vi "Example-ITC.vi"() -> ()   [LabVIEW 2013, in "Mercury iXX.lvlib"]
uses:
  <instrlib>/Mercury iXX/Mercury iXX.lvlib
  <instrlib>/Mercury iXX/Public/Controls/Unit String.ctl
  <instrlib>/Mercury iXX/Public/Libraries/Temperature/Controls/Temperature Device (Read).ctl
  <instrlib>/Mercury iXX/Public/Controls/Manufacturing Data.ctl
  <instrlib>/Mercury iXX/Public/Libraries/Temperature/Controls/Temperature Sensor Type.ctl
  <instrlib>/Mercury iXX/Public/Libraries/Temperature/Controls/Excitation Cluster.ctl
  <instrlib>/Mercury iXX/Public/Libraries/Temperature/Controls/Excitation Type.ctl
  <instrlib>/Mercury iXX/Public/Libraries/Temperature/Controls/Calibration Cluster.ctl
  <instrlib>/Mercury iXX/Public/Libraries/Temperature/Controls/Calibration Interpolation.ctl
  <instrlib>/Mercury iXX/Public/Libraries/Temperature/Controls/Loop Cluster.ctl
  <instrlib>/Mercury iXX/Public/Libraries/Temperature/Controls/Temperature Signals Cluster.ctl
  <instrlib>/Mercury iXX/Public/Libraries/Heater/Controls/Heater Device (Read).ctl
  <instrlib>/Mercury iXX/Public/Libraries/Heater/Controls/Heater Signals Cluster.ctl
  <instrlib>/Mercury iXX/Public/Libraries/Auxiliary/Controls/AUX Device (Read).ctl
  <instrlib>/Mercury iXX/Public/Libraries/Auxiliary/Controls/AUX Signals (Read).ctl
  <instrlib>/Mercury iXX/Public/Libraries/Pressure/Controls/Pressure Device (Read).ctl
  <instrlib>/Mercury iXX/Public/Libraries/Pressure/Controls/Pressure Sensor Type.ctl
  <instrlib>/Mercury iXX/Public/Libraries/Pressure/Controls/Calibration Cluster.ctl
  <instrlib>/Mercury iXX/Public/Libraries/Pressure/Controls/Calibration Interpolation.ctl
  <instrlib>/Mercury iXX/Public/Libraries/Pressure/Controls/Loop Cluster.ctl
  <instrlib>/Mercury iXX/Public/Libraries/Pressure/Controls/Pressure Signals Cluster.ctl
  <instrlib>/Mercury iXX/Public/Libraries/Flow/Controls/Flow Device (Read).ctl
  <instrlib>/Mercury iXX/Public/Libraries/Flow/Controls/Flow Signals Cluster.ctl
  <instrlib>/Mercury iXX/Public/Controls/Comms Transport Layer.ctl
  <instrlib>/Mercury iXX/Public/Controls/ISOBus Address.ctl
  <instrlib>/Mercury iXX/Public/Libraries/System/Open/Open System.vi
  <instrlib>/Mercury iXX/Public/Libraries/System/Read/Catalogue (Read).vi
  <instrlib>/Mercury iXX/Public/Libraries/System/Read/Display Automatic Dimming (Read).vi
  <instrlib>/Mercury iXX/Public/Libraries/System/Read/Display Automatic Dimming Time (Read).vi
  <instrlib>/Mercury iXX/Public/Libraries/System/Read/Display Brightness (Read).vi
  <instrlib>/Mercury iXX/Public/Libraries/System/Read/Date (Read).vi
  <instrlib>/Mercury iXX/Public/Libraries/System/Read/Time (Read).vi
  <instrlib>/Mercury iXX/Public/Libraries/System/Read/DateTime (Read).vi
  <instrlib>/Mercury iXX/Public/Libraries/System/Read/HVer (Read).vi
  <instrlib>/Mercury iXX/Public/Libraries/System/Read/FVer (Read).vi
  <instrlib>/Mercury iXX/Public/Libraries/System/Read/Serial Number (Read).vi
  <instrlib>/Mercury iXX/Public/Libraries/System/Read/Flash Space (Read).vi
  <instrlib>/Mercury iXX/Public/Libraries/System/Read/Mode (Read).vi
  <instrlib>/Mercury iXX/Public/Libraries/Auxiliary/Open/Open Auxiliary Device.vi
  <instrlib>/Mercury iXX/Public/Libraries/Auxiliary/Configuration/Read/Aux Device (Read).vi
  <instrlib>/Mercury iXX/Public/Libraries/Auxiliary/Configuration/Read/Serial Number (Read).vi
  <instrlib>/Mercury iXX/Public/Libraries/Auxiliary/Configuration/Read/Minimum Gas Flow (Read).vi
  <instrlib>/Mercury iXX/Public/Libraries/Auxiliary/Configuration/Read/Gas Flow Scaling (Read).vi
  <instrlib>/Mercury iXX/Public/Libraries/Auxiliary/Configuration/Read/Temperature Error Sensitivity (Read).vi
  <instrlib>/Mercury iXX/Public/Libraries/Auxiliary/Configuration/Read/Temperature Error Voltage Sensitivity (Read).vi
  <instrlib>/Mercury iXX/Public/Libraries/Auxiliary/Configuration/Read/Valve Gearing (Read).vi
  <instrlib>/Mercury iXX/Public/Libraries/Auxiliary/Configuration/Read/Stepper Speed (Read).vi
  <instrlib>/Mercury iXX/Public/Libraries/Auxiliary/Signals/Read/Position (Read).vi
  <instrlib>/Mercury iXX/Public/Libraries/Auxiliary/Signals/Read/Percent Open (Read).vi
  <instrlib>/Mercury iXX/Public/Libraries/Pressure/Open/Open Pressure Device.vi
  <instrlib>/Mercury iXX/Public/Libraries/Pressure/Configuration/Read/Pressure Device (Read).vi
  <instrlib>/Mercury iXX/Public/Libraries/Pressure/Configuration/Read/Nickname (Read).vi
  <instrlib>/Mercury iXX/Public/Libraries/Pressure/Signals/Read/Current (Read).vi
  <instrlib>/Mercury iXX/Public/Libraries/Pressure/Signals/Read/Voltage (Read).vi
  <instrlib>/Mercury iXX/Public/Libraries/Heater/Open/Open Heater Device.vi
  <instrlib>/Mercury iXX/Public/Libraries/Heater/Configuration/Read/Heater Device (Read).vi
  <instrlib>/Mercury iXX/Public/Libraries/Heater/Configuration/Read/Nickname (Read).vi
  <instrlib>/Mercury iXX/Public/Libraries/Heater/Configuration/Read/Serial Number (Read).vi
  <instrlib>/Mercury iXX/Public/Libraries/Heater/Configuration/Read/Voltage Limit (Read).vi
  <instrlib>/Mercury iXX/Public/Libraries/Heater/Configuration/Read/Nominal Resistance (Read).vi
  <instrlib>/Mercury iXX/Public/Libraries/Heater/Configuration/Read/Maximum Power (Read).vi
  <instrlib>/Mercury iXX/Public/Libraries/Heater/Signals/Read/Voltage (Read).vi
  <instrlib>/Mercury iXX/Public/Libraries/Heater/Signals/Read/Power (Read).vi
  <instrlib>/Mercury iXX/Public/Libraries/Heater/Signals/Read/Current (Read).vi
  <instrlib>/Mercury iXX/Public/Libraries/Temperature/Open/Open Temperature Device.vi
  <instrlib>/Mercury iXX/Public/Libraries/Temperature/Configuration/Read/Serial Number (Read).vi
  <instrlib>/Mercury iXX/Public/Libraries/Temperature/Configuration/Read/Nickname (Read).vi
  <instrlib>/Mercury iXX/Public/Libraries/Temperature/Configuration/Read/Excitation Magnitude (Read).vi
  <instrlib>/Mercury iXX/Public/Libraries/Temperature/Configuration/Read/Temperature Sensor (Read).vi
  <instrlib>/Mercury iXX/Public/Libraries/Temperature/Configuration/Read/Excitation Type (Read).vi
  <instrlib>/Mercury iXX/Public/Libraries/Temperature/Configuration/Read/Calibration Hot Limit (Read).vi
  <instrlib>/Mercury iXX/Public/Libraries/Temperature/Configuration/Read/Calibration Cold Limit (Read).vi
  <instrlib>/Mercury iXX/Public/Libraries/Temperature/Signals/Read/Temperature (Read).vi
  <instrlib>/Mercury iXX/Public/Libraries/Temperature/Configuration/Read/Temperature Device (Read).vi
  <instrlib>/Mercury iXX/Public/Libraries/Control Loop/Configuration/Read/Control Loop (Read).vi
  <instrlib>/Mercury iXX/Public/Libraries/System/Set/DateTime (Set).vi
  <instrlib>/Mercury iXX/Public/Libraries/Pressure.lvlib
  <instrlib>/Mercury iXX/Public/Libraries/System.lvlib
  <instrlib>/Mercury iXX/Public/Libraries/Auxiliary.lvlib
  <instrlib>/Mercury iXX/Public/Libraries/Control Loop.lvlib
  <instrlib>/Mercury iXX/Public/Libraries/Heater.lvlib
  <instrlib>/Mercury iXX/Public/Libraries/Temperature.lvlib
  <instrlib>/Mercury iXX/Public/Libraries/Flow/Open/Open Flow Device.vi
  <instrlib>/Mercury iXX/Public/Libraries/Flow.lvlib
  <instrlib>/Mercury iXX/Public/Libraries/Flow/Configuration/Read/Flow Device (Read).vi
  <instrlib>/Mercury iXX/Public/Libraries/Flow/Configuration/Read/Maximum Power (Read).vi
  <instrlib>/Mercury iXX/Public/Libraries/Flow/Configuration/Read/Fastcool Mode (Read).vi
  <instrlib>/Mercury iXX/Public/Libraries/Flow/Signals/Read/Voltage (Read).vi
  <instrlib>/Mercury iXX/Public/Libraries/Flow/Signals/Read/Current (Read).vi
panel:
  in  "Mercury Functions":T1(tab)
  out "time stamp":timestamp=timestamp(3542718986 s since 1904-01-01)
  out "Free Space":i32=166152 caption="Free Space (KB)"
  out "Set Date Response":string="VALID"
  out "String":string="NORM" caption="User Mode"
  out "Date":string="2016:04:05"
  out "Time":string="11:36:26"
  out "Hardware Version":string="65"
  out "Firmware Version":string="2.2.6.20"
  out "Serial Number":string="153350063"
  out "Devices":string[](array[string])=["DB3.L1:LVL", "GRPX:PSU", "GRPY:PSU", "GRPZ:PSU", "MB1.T1:TEMP", "PSU.M1:PSU", "PSU.M2:PSU", "PSU.M3:PSU"]
  out "S/W Version(s)":string[](array[string])=["2.2.6.20\n"]
  out "Serial Number(s)":string[](array[string])=["153350063"]
  out "# of Instruments":i32=1
  out "Automatic Dimming":string="OFF"
  out "Dimming Time":string="5"
  out "Display Brightness":string="100"
  in  "ITC IP Address":string="130.49.180.102"
  out "Excitation Magnitude":dbl
  out "Sensor Type":string="DUM"
  out "Excitation Type":string="UNIP"
  out "Hot Limit":dbl=1000.0
  out "H Unit":T2="K"
  out "Cold Limit":dbl=1000.0
  out "C Unit":T2="K"
  out "Unit":T2
  out "Voltage":dbl
  out "V Unit":T2="A"
  out "Temperature":dbl
  out "T Unit":T2="K"
  out "Temperature Device Settings":T3={"Manufacturing"={"Hardware Version"="65", "Firmware Version"="2.2", "Serial Number"="153350063"}, "Temperature Sensor Type"="DUM", "Excitation"={"Excitation Type"="UNIP", "Magnitude"="0"}, "Calibration"={"Filename"="None", "Interpolation"="LIN", "Scaling Factor"="1", "Offset Factor"="0", "Hot Limit"="1000.00K", "Cold Limit"="1000.00K", "Last Calibration"="", "Reference"="Internal"}, "Control Loop"={"Heater"="", "Auxiliary"="", "Heater Auto"="", "Percentage Heat"="", "Temperature Set Point"="", "PID Auto (from file)"="", "P Value"="", "I Value"="", "D Value"="", "Auto PID Table Filename"="", "Flow Auto"="", "Target Heater Table"="", "Sweep mode"="", "Sweep Table Filename"="", "Percentage Flow"=""}, "Temperature Signals"={"Voltage"="0.0000V", "Current"="0.0000A", "Power"="N/A", "Resistance"="", "Temperature"="0.0000K", "Sensitivity"="", "Reference"=""}, "Nickname"="MB1.T1", "Status"="0"}
  out "Temp S/N":string="153350063"
  out "T Nickname":string="MB1.T1"
  out "T Loop Details":T10
  out "Heater Device Settings":T12={"Manufacturing"={"Hardware Version"="", "Firmware Version"="", "Serial Number"=""}, "Nickname"="", "Voltage Limit"="", "Nominal Resistance"="", "Maximum Power"="", "Heater Signals"={"Voltage"="", "Current"="", "Power"=""}, "Status"="DEV"}
  out "Htr C Unit":T2
  out "Htr P Unit":T2
  out "Htr V Unit":T2
  out "Htr Current":dbl
  out "Htr Power":dbl
  out "Htr Voltage":dbl
  out "Power Unit":T2
  out "Volt Unit":T2
  out "Res Unit":T2
  out "Maximum Power":dbl
  out "Htr Resistance":dbl
  out "Htr Voltage Limit":dbl
  out "Htr S/N":string="STAT:DEV:MB0.H1:N/A"
  out "Htr Nickname":string="STAT:DEV:MB0.H1:N/A"
  out "Auxiliary Device Details":T14 {"Signals"."% Open" min=0.0 max=100.0 step=0.1 format="%.4f"; "Signals"."Position" max=20.0 step=1.0 format="%.4f"; "Speed" max=7 step=1; "Gear" max=7 step=1; "Temp V Err" min=0.0 max=20.0 step=0.1; "Temp Err" min=0.0 max=20.0 step=0.1; "Scaling Factor" min=0.0 max=99.0 step=0.1; "Min Flow" min=0.0 max=20.0 step=0.1}
  out "Aux S/N":string
  out "Min Flow":dbl=-inf caption="Minimum Gas Flow" format="%#.1f"
  out "Scaling Factor":dbl=-inf caption="Gas Flow Scaling Factor" format="%#.1f"
  out "Temp Err":dbl=-inf caption="Temperature Error Sensitivity" format="%#.1f"
  out "Temp V Err":dbl=-inf caption="Temperature Voltage Error Sensitivity" format="%#.1f"
  out "Gear":u32 caption="Valve Gearing"
  out "Speed":u32 caption="Stepper Speed"
  out "Unit 2":T2="ERR"
  out "Unit 3":T2="ERR"
  out "Unit 4":T2="ERR"
  out "Unit 5":T2="ERR"
  out "Unit 6":T2="ERR"
  out "Unit 7":T2="ERR"
  out "Position":u32
  out "% Open":dbl=-inf caption="Percentage Open (%)"
  out "Unit":T2="ERR"
  out "Unit":T2="ERR"
  out "Pressure Device":T16={"Manufacturing"={"Hardware Version"="", "Firmware Version"="", "Serial Number"=""}, "Temperature Sensor Type"="", "Calibration"={"Filename"="", "Interpolation"="", "Scaling Factor"="", "Offset Factor"="", "High Limit"="", "Low Limit"="", "Last Calibration"=""}, "Control Loop"={"Heater"="", "Auxiliary"="", "Heater Auto"="", "Percentage Heat"="", "Pressure Set Point"="", "PID Auto (from file)"="", "P Value"="", "I Value"="", "D Value"="", "Auto PID Table Filename"="", "Flow Auto"="", "Target Heater Table"="", "Sweep mode"="", "Sweep Table Filename"="", "Percentage Flow"=""}, "Pressure Signals"={"Voltage"="", "Current"="", "Power"="", "Pressure"=""}, "Nickname"="", "Status"="DEV"}
  out "Nickname":string="STAT:DEV:DB6.P1:N/A"
  out "Current":dbl
  out "Voltage":dbl
  out "Flow Device":T22
  out "Maximum Power 2":dbl
  out "Fastcool Mode":string
  out "Current 2":dbl
  out "Voltage 2":dbl
  # "ITC"
  # "101, 102, 67"
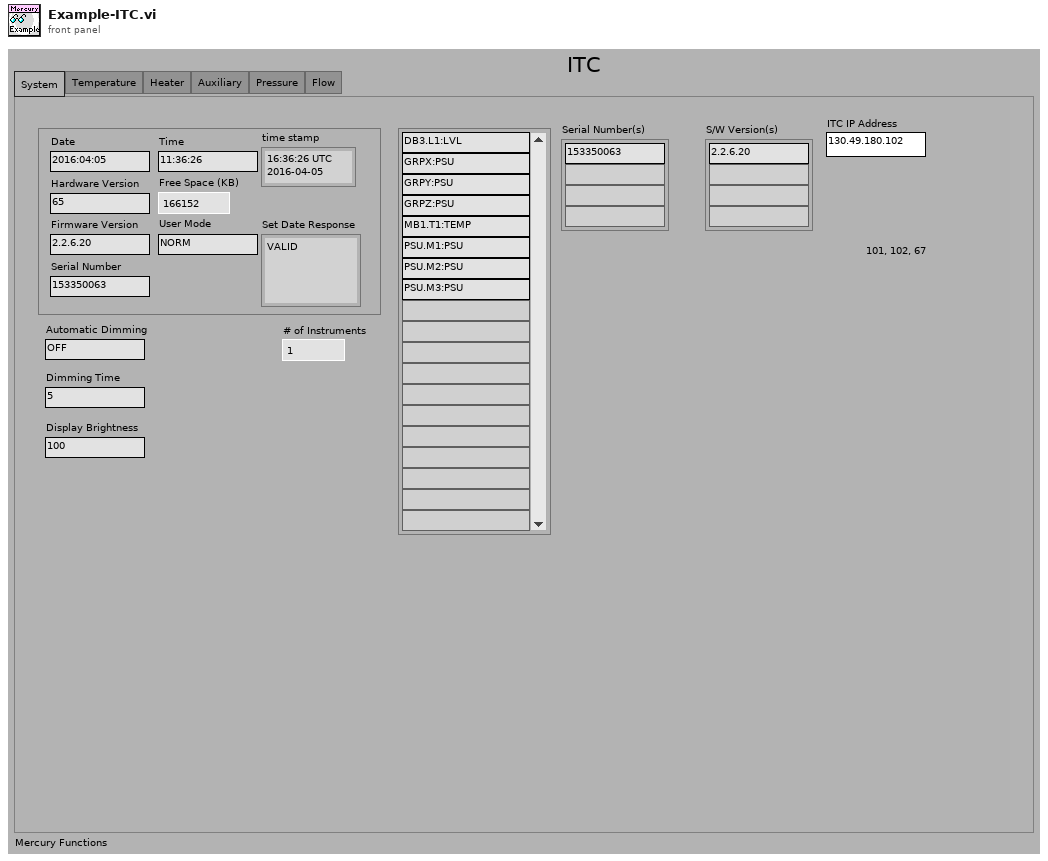
[diagram p1: front panel]
types:
  T1 = enum32{"System", "Temperature", "Heater", "Auxiliary", "Pressure", "Flow"}
  T2 = typedef "Mercury iXX.lvlib/Unit String.ctl" = string
  T3 = typedef "Mercury iXX.lvlib/Temperature.lvlib/Temperature Device (Read).ctl" = cluster{"Manufacturing":T4, "Temperature Sensor Type":T5, "Excitation":T6, "Calibration":T8, "Control Loop":T10, "Temperature Signals":T11, "Nickname":string, "Status":string}
  T4 = typedef "Mercury iXX.lvlib/Manufacturing Data.ctl" = cluster{"Hardware Version":string, "Firmware Version":string, "Serial Number":string}
  T5 = typedef "Mercury iXX.lvlib/Temperature.lvlib/Temperature Sensor Type.ctl" = string
  T6 = typedef "Mercury iXX.lvlib/Temperature.lvlib/Excitation Cluster.ctl" = cluster{"Excitation Type":T7, "Magnitude":string}
  T7 = typedef "Mercury iXX.lvlib/Temperature.lvlib/Excitation Type.ctl" = string
  T8 = typedef "Mercury iXX.lvlib/Temperature.lvlib/Calibration Cluster.ctl" = cluster{"Filename":string, "Interpolation":T9, "Scaling Factor":string, "Offset Factor":string, "Hot Limit":string, "Cold Limit":string, "Last Calibration":string, "Reference":string}
  T9 = typedef "Mercury iXX.lvlib/Temperature.lvlib/Calibration Interpolation.ctl" = string
  T10 = typedef "Mercury iXX.lvlib/Temperature.lvlib/Loop Cluster.ctl" = cluster{"Heater":string, "Auxiliary":string, "Heater Auto":string, "Percentage Heat":string, "Temperature Set Point":string, "PID Auto (from file)":string, "P Value":string, "I Value":string, "D Value":string, "Auto PID Table Filename":string, "Flow Auto":string, "Target Heater Table":string, "Sweep mode":string, "Sweep Table Filename":string, "Percentage Flow":string}
  T11 = typedef "Mercury iXX.lvlib/Temperature.lvlib/Temperature Signals Cluster.ctl" = cluster{"Voltage":string, "Current":string, "Power":string, "Resistance":string, "Temperature":string, "Sensitivity":string, "Reference":string}
  T12 = typedef "Mercury iXX.lvlib/Heater.lvlib/Heater Device (Read).ctl" = cluster{"Manufacturing":T4, "Nickname":string, "Voltage Limit":string, "Nominal Resistance":string, "Maximum Power":string, "Heater Signals":T13, "Status":string}
  T13 = typedef "Mercury iXX.lvlib/Heater.lvlib/Heater Signals Cluster.ctl" = cluster{"Voltage":string, "Current":string, "Power":string}
  T14 = typedef "Mercury iXX.lvlib/Auxiliary.lvlib/AUX Device (Read).ctl" = cluster{"Manufacturing":T4, "Min Flow":dbl, "Scaling Factor":dbl, "Temp Err":dbl, "Temp V Err":dbl, "Gear":u32, "Speed":u32, "Signals":T15, "Nickname":string, "Status":string}
  T15 = typedef "Mercury iXX.lvlib/Auxiliary.lvlib/AUX Signals (Read).ctl" = cluster{"Position":dbl, "% Open":dbl, "I0":string, "I1":string, "I2":string, "I3":string, "O0":string, "O1":string, "O2":string, "O3":string}
  T16 = typedef "Mercury iXX.lvlib/Pressure.lvlib/Pressure Device (Read).ctl" = cluster{"Manufacturing":T4, "Temperature Sensor Type":T17, "Calibration":T18, "Control Loop":T20, "Pressure Signals":T21, "Nickname":string, "Status":string}
  T17 = typedef "Mercury iXX.lvlib/Pressure.lvlib/Pressure Sensor Type.ctl" = string
  T18 = typedef "Mercury iXX.lvlib/Pressure.lvlib/Calibration Cluster.ctl" = cluster{"Filename":string, "Interpolation":T19, "Scaling Factor":string, "Offset Factor":string, "High Limit":string, "Low Limit":string, "Last Calibration":string}
  T19 = typedef "Mercury iXX.lvlib/Pressure.lvlib/Calibration Interpolation.ctl" = string
  T20 = typedef "Mercury iXX.lvlib/Pressure.lvlib/Loop Cluster.ctl" = cluster{"Heater":string, "Auxiliary":string, "Heater Auto":string, "Percentage Heat":string, "Pressure Set Point":string, "PID Auto (from file)":string, "P Value":string, "I Value":string, "D Value":string, "Auto PID Table Filename":string, "Flow Auto":string, "Target Heater Table":string, "Sweep mode":string, "Sweep Table Filename":string, "Percentage Flow":string}
  T21 = typedef "Mercury iXX.lvlib/Pressure.lvlib/Pressure Signals Cluster.ctl" = cluster{"Voltage":string, "Current":string, "Power":string, "Pressure":string}
  T22 = typedef "Mercury iXX.lvlib/Flow.lvlib/Flow Device (Read).ctl" = cluster{"Manufacturing":T4, "Nickname":string, "Voltage Limit":string, "Nominal Resistance":string, "Maximum Power":string, "Flow Signals":T23, "Status":string, "Fastcool Mode":string}
  T23 = typedef "Mercury iXX.lvlib/Flow.lvlib/Flow Signals Cluster.ctl" = cluster{"Voltage":string, "Current":string, "Power":string, "Flow":string}
  T24 = typedef "Mercury iXX.lvlib/ISOBus Address.ctl" = i32
  T25 = typedef "Mercury iXX.lvlib/Comms Transport Layer.ctl" = enum16{"Ethernet TCP/IP", "USB", "ISOBus - RS-232", "GPIB"}
  T26 = typedef "Mercury iXX.lvlib/Mercury Reference.ctl" = cluster{"Comms":refnum<visa-resource-name>, "Device ID":string[], "Comms Layer":T25, "Command":string, "Query reference":T27}
  T27 = typedef "Mercury iXX.lvlib/Query Dynamic Reference.ctl" = refnum<vi>
  T28 = typedef "Mercury iXX.lvlib/System.lvlib/User Mode.ctl" = string
  T29 = typedef "Mercury iXX.lvlib/Response String.ctl" = string
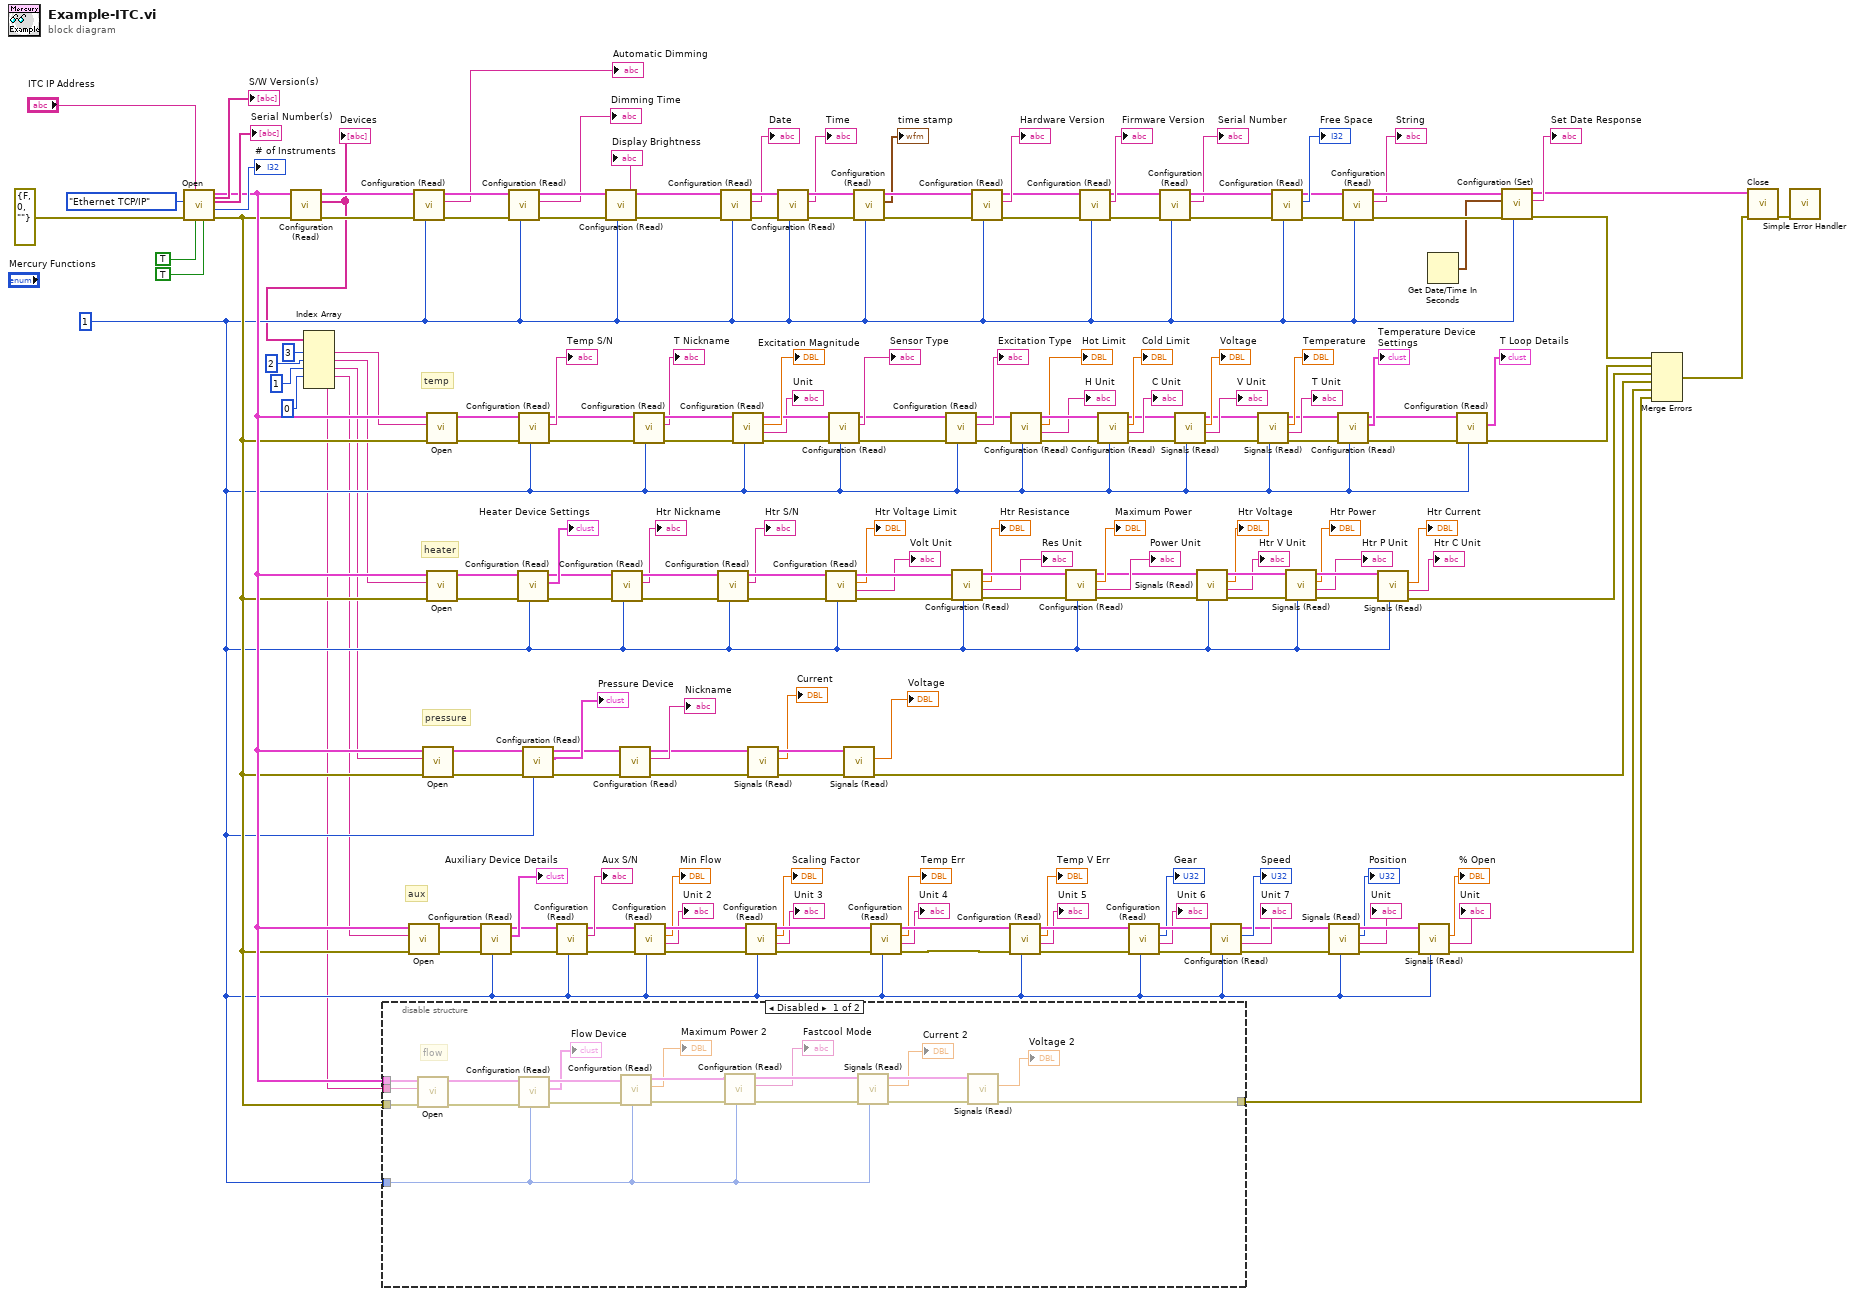
[diagram p0: block diagram]
diagram:
  w11 = T24 1 ("ISOBUS address")
  # "aux"
  # "pressure"
  # "heater"
  # "temp"
  n1 = call-poly <instrlib>:"Open.vi"("Clear Previous Connections (False)"=TRUE ("Clear Previous Connections (True)"), "ID Query (True)"=TRUE, "IP Address"="ITC IP Address", "error in (no error)"=errorcluster {"status"=FALSE, "code"=0, "source"=""}, "Comms Layer"=Comms_Transport_Layer."Ethernet TCP/IP") -> ("error out"=w12:errorcluster, "# of Instruments"=→"# of Instruments":i32, "Serial Number(s)"=→"Serial Number(s)":string[], "Mercury Reference Out"=w13:T26, "S/W Version(s)"=→"S/W Version(s)":string[])  [unwired: 2 in]
  n2 = call-poly <instrlib>:"Configuration (Read).vi"("error in"=w12, "Mercury Reference In"=w13) -> ("error out"=w34:errorcluster, "Devices"=w9:string[], "Mercury Reference Out"=w33:T26)  [unwired: 1 in, 6 out]
  "Devices" <- w9
  n3 = Index Array(array=w9, index #1=3 ("index"), index #2=2 ("index"), index #3=1 ("index"), index #4=0 ("index")) -> (element #1=w7:string, element #2=w6:string, element #3=w5:string, element #4=w4:string, element #5=w1:string)  [unwired: 1 in]
  n4 = disable-structure shown="Disabled" {
    disable-tunnel: w13 -> [w203 _]
    disable-tunnel: w12 -> [w202 _]
    disable-tunnel: w11 -> [w201 _]
    disable-tunnel: [w195 _] -> w10
    disable-tunnel: w1 -> [w189 _]
    frame Disabled {
      # "flow"
      n5 = call-poly <instrlib>:"Open.vi"("error in (no error)"=w202, "Device Identifier"=w189, "Mercury Reference In"=w203) -> ("error out"=w204:errorcluster, "Mercury Reference Out"=w200:T26)  [unwired: 7 out]
      n6 = call-poly <instrlib>:"Configuration (Read).vi"("ISOBUS address"=w201, "error in"=w204, "Mercury Reference In"=w200) -> ("error out"=w206:errorcluster, "Device Details"=→"Flow Device":T22, "Mercury Reference Out"=w199:T26)  [unwired: 6 out]
      n7 = call-poly <instrlib>:"Configuration (Read).vi"("ISOBUS address"=w201, "error in"=w206, "Mercury Reference In"=w199) -> ("error out"=w205:errorcluster, "Maximum Power"=→"Maximum Power 2":dbl, "Mercury Reference Out"=w198:T26)  [unwired: 6 out]
      n8 = call-poly <instrlib>:"Configuration (Read).vi"("ISOBUS address"=w201, "error in"=w205, "Mercury Reference In"=w198) -> ("error out"=w208:errorcluster, "Fastcool Mode"=→"Fastcool Mode":string, "Mercury Reference Out"=w197:T26)  [unwired: 6 out]
      n9 = call-poly <instrlib>:"Signals (Read).vi"("ISOBUS address"=w201, "error in"=w208, "Mercury Reference In"=w197) -> ("error out"=w207:errorcluster, "Current"=→"Current 2":dbl, "Mercury Reference Out"=w196:T26)  [unwired: 6 out]
      n10 = call-poly <instrlib>:"Signals (Read).vi"("error in"=w207, "Mercury Reference In"=w196) -> ("error out"=w195:errorcluster, "Voltage"=→"Voltage 2":dbl)  [unwired: 1 in, 7 out]
    }
    frame Enabled {
    }
  }
  n11 = call-poly <instrlib>:"Open.vi"("error in (no error)"=w12, "Device Identifier"=w4, "Mercury Reference In"=w13) -> ("error out"=w95:errorcluster, "Mercury Reference Out"=w94:T26)  [unwired: 7 out]
  n12 = call-poly <instrlib>:"Configuration (Read).vi"("ISOBUS address"=w11, "error in"=w34, "Mercury Reference In"=w33) -> ("error out"=w41:errorcluster, "Automatic Dimming"=→"Automatic Dimming":string, "Mercury Reference Out"=w40:T26)  [unwired: 6 out]
  n13 = call-poly <instrlib>:"Open.vi"("error in (no error)"=w12, "Device Identifier"=w5, "Mercury Reference In"=w13) -> ("error out"=w29:errorcluster, "Mercury Reference Out"=w28:T26)  [unwired: 7 out]
  n14 = call-poly <instrlib>:"Open.vi"("error in (no error)"=w12, "Device Identifier"=w7, "Mercury Reference In"=w13) -> ("error out"=w44:errorcluster, "Mercury Reference Out"=w43:T26)  [unwired: 7 out]
  n15 = call-poly <instrlib>:"Open.vi"("error in (no error)"=w12, "Device Identifier"=w6, "Mercury Reference In"=w13) -> ("error out"=w139:errorcluster, "Mercury Reference Out"=w140:T26)  [unwired: 7 out]
  n16 = call-poly <instrlib>:"Configuration (Read).vi"("ISOBUS address"=w11, "error in"=w95, "Mercury Reference In"=w94) -> ("error out"=w91:errorcluster, "Auxiliary Device Details"=→"Auxiliary Device Details":T14, "Mercury Reference Out"=w92:T26)  [unwired: 6 out]
  n17 = call-poly <instrlib>:"Configuration (Read).vi"("ISOBUS address"=w11, "error in"=w41, "Mercury Reference In"=w40) -> ("error out"=w38:errorcluster, "Dimming Time"=→"Dimming Time":string, "Mercury Reference Out"=w39:T26)  [unwired: 6 out]
  n18 = call-poly <instrlib>:"Configuration (Read).vi"("ISOBUS address"=w11, "error in"=w139, "Mercury Reference In"=w140) -> ("error out"=w108:errorcluster, "Device Details"=→"Heater Device Settings":T12, "Mercury Reference Out"=w109:T26)  [unwired: 6 out]
  n19 = call-poly <instrlib>:"Configuration (Read).vi"("ISOBUS address"=w11, "error in"=w44, "Mercury Reference In"=w43) -> ("error out"=w170:errorcluster, "Serial Number"=→"Temp S/N":string, "Mercury Reference Out"=w171:T26)  [unwired: 6 out]
  n20 = call-poly <instrlib>:"Configuration (Read).vi"("ISOBUS address"=w11, "error in"=w29, "Mercury Reference In"=w28) -> ("error out"=w27:errorcluster, "Device Details"=→"Pressure Device":T16, "Mercury Reference Out"=w26:T26)  [unwired: 6 out]
  n21 = call-poly <instrlib>:"Configuration (Read).vi"("ISOBUS address"=w11, "error in"=w91, "Mercury Reference In"=w92) -> ("error out"=w88:errorcluster, "Serial Number"=→"Aux S/N":string, "Mercury Reference Out"=w89:T26)  [unwired: 6 out]
  n22 = call-poly <instrlib>:"Configuration (Read).vi"("ISOBUS address"=w11, "error in"=w38, "Mercury Reference In"=w39) -> ("error out"=w32:errorcluster, "Display Brightness"=→"Display Brightness":string, "Mercury Reference Out"=w31:T26)  [unwired: 6 out]
  n23 = call-poly <instrlib>:"Configuration (Read).vi"("ISOBUS address"=w11, "error in"=w108, "Mercury Reference In"=w109) -> ("error out"=w106:errorcluster, "Nickname"=→"Htr Nickname":string, "Mercury Reference Out"=w107:T26)  [unwired: 6 out]
  n24 = call-poly <instrlib>:"Configuration (Read).vi"("error in"=w27, "Mercury Reference In"=w26) -> ("error out"=w22:errorcluster, "Nickname"=→"Nickname":string, "Mercury Reference Out"=w21:T26)  [unwired: 1 in, 6 out]
  n25 = call-poly <instrlib>:"Configuration (Read).vi"("ISOBUS address"=w11, "error in"=w170, "Mercury Reference In"=w171) -> ("error out"=w168:errorcluster, "Nickname"=→"T Nickname":string, "Mercury Reference Out"=w169:T26)  [unwired: 6 out]
  n26 = call-poly <instrlib>:"Configuration (Read).vi"("ISOBUS address"=w11, "error in"=w88, "Mercury Reference In"=w89) -> ("error out"=w86:errorcluster, "Unit"=→"Unit 2":T2, "Min Flow"=→"Min Flow":dbl, "Mercury Reference Out"=w87:T26)  [unwired: 5 out]
  n27 = call-poly <instrlib>:"Configuration (Read).vi"("ISOBUS address"=w11, "error in"=w106, "Mercury Reference In"=w107) -> ("error out"=w136:errorcluster, "Serial Number"=→"Htr S/N":string, "Mercury Reference Out"=w137:T26)  [unwired: 6 out]
  n28 = call-poly <instrlib>:"Configuration (Read).vi"("ISOBUS address"=w11, "error in"=w32, "Mercury Reference In"=w31) -> ("error out"=w187:errorcluster, "Date"=→"Date":string, "Mercury Reference Out"=w188:T26)  [unwired: 6 out]
  n29 = call-poly <instrlib>:"Configuration (Read).vi"("ISOBUS address"=w11, "error in"=w168, "Mercury Reference In"=w169) -> ("error out"=w165:errorcluster, "Unit"=→"Unit":T2, "Excitation Magnitude"=→"Excitation Magnitude":dbl, "Mercury Reference Out"=w166:T26)  [unwired: 5 out]
  n30 = call-poly <instrlib>:"Configuration (Read).vi"("ISOBUS address"=w11, "error in"=w86, "Mercury Reference In"=w87) -> ("error out"=w84:errorcluster, "Unit"=→"Unit 3":T2, "Scaling Factor"=→"Scaling Factor":dbl, "Mercury Reference Out"=w85:T26)  [unwired: 5 out]
  n31 = call-poly <instrlib>:"Signals (Read).vi"("error in"=w22, "Mercury Reference In"=w21) -> ("error out"=w24:errorcluster, "Current"=→"Current":dbl, "Mercury Reference Out"=w23:T26)  [unwired: 1 in, 6 out]
  n32 = call-poly <instrlib>:"Configuration (Read).vi"("ISOBUS address"=w11, "error in"=w187, "Mercury Reference In"=w188) -> ("error out"=w185:errorcluster, "Time"=→"Time":string, "Mercury Reference Out"=w186:T26)  [unwired: 6 out]
  n33 = call-poly <instrlib>:"Configuration (Read).vi"("ISOBUS address"=w11, "error in"=w136, "Mercury Reference In"=w137) -> ("error out"=w135:errorcluster, "Unit"=→"Volt Unit":T2, "Voltage Limit"=→"Htr Voltage Limit":dbl, "Mercury Reference Out"=w132:T26)  [unwired: 5 out]
  n34 = call-poly <instrlib>:"Configuration (Read).vi"("ISOBUS address"=w11, "error in"=w165, "Mercury Reference In"=w166) -> ("error out"=w162:errorcluster, "Sensor Type"=→"Sensor Type":T5, "Mercury Reference Out"=w163:T26)  [unwired: 6 out]
  n35 = call-poly <instrlib>:"Signals (Read).vi"("error in"=w24, "Mercury Reference In"=w23) -> ("error out"=w15:errorcluster, "Voltage"=→"Voltage":dbl)  [unwired: 1 in, 7 out]
  n36 = call-poly <instrlib>:"Configuration (Read).vi"("ISOBUS address"=w11, "error in"=w185, "Mercury Reference In"=w186) -> ("error out"=w183:errorcluster, "time stamp"=→"time stamp":timestamp, "Mercury Reference Out"=w184:T26)  [unwired: 6 out]
  n37 = call-poly <instrlib>:"Configuration (Read).vi"("ISOBUS address"=w11, "error in"=w84, "Mercury Reference In"=w85) -> ("error out"=w82:errorcluster, "Unit"=→"Unit 4":T2, "Temp Err"=→"Temp Err":dbl, "Mercury Reference Out"=w83:T26)  [unwired: 5 out]
  n38 = call-poly <instrlib>:"Configuration (Read).vi"("ISOBUS address"=w11, "error in"=w162, "Mercury Reference In"=w163) -> ("error out"=w160:errorcluster, "Excitation Type"=→"Excitation Type":T7, "Mercury Reference Out"=w159:T26)  [unwired: 6 out]
  n39 = call-poly <instrlib>:"Configuration (Read).vi"("ISOBUS address"=w11, "error in"=w135, "Mercury Reference In"=w132) -> ("error out"=w134:errorcluster, "Unit"=→"Res Unit":T2, "Nominal Resistance"=→"Htr Resistance":dbl, "Mercury Reference Out"=w133:T26)  [unwired: 5 out]
  n40 = call-poly <instrlib>:"Configuration (Read).vi"("ISOBUS address"=w11, "error in"=w183, "Mercury Reference In"=w184) -> ("error out"=w45:errorcluster, "Hardware Version"=→"Hardware Version":string, "Mercury Reference Out"=w46:T26)  [unwired: 6 out]
  n41 = call-poly <instrlib>:"Configuration (Read).vi"("ISOBUS address"=w11, "error in"=w82, "Mercury Reference In"=w83) -> ("error out"=w80:errorcluster, "Unit"=→"Unit 5":T2, "Temp V Err"=→"Temp V Err":dbl, "Mercury Reference Out"=w81:T26)  [unwired: 5 out]
  n42 = call-poly <instrlib>:"Configuration (Read).vi"("ISOBUS address"=w11, "error in"=w160, "Mercury Reference In"=w159) -> ("error out"=w158:errorcluster, "Unit"=→"H Unit":T2, "Hot Limit"=→"Hot Limit":dbl, "Mercury Reference Out"=w157:T26)  [unwired: 5 out]
  n43 = call-poly <instrlib>:"Configuration (Read).vi"("ISOBUS address"=w11, "error in"=w134, "Mercury Reference In"=w133) -> ("error out"=w124:errorcluster, "Unit"=→"Power Unit":T2, "Maximum Power"=→"Maximum Power":dbl, "Mercury Reference Out"=w125:T26)  [unwired: 5 out]
  n44 = call-poly <instrlib>:"Configuration (Read).vi"("ISOBUS address"=w11, "error in"=w45, "Mercury Reference In"=w46) -> ("error out"=w47:errorcluster, "Firmware Version"=→"Firmware Version":string, "Mercury Reference Out"=w48:T26)  [unwired: 6 out]
  n45 = call-poly <instrlib>:"Configuration (Read).vi"("ISOBUS address"=w11, "error in"=w158, "Mercury Reference In"=w157) -> ("error out"=w150:errorcluster, "Unit"=→"C Unit":T2, "Cold Limit"=→"Cold Limit":dbl, "Mercury Reference Out"=w151:T26)  [unwired: 5 out]
  n46 = call-poly <instrlib>:"Configuration (Read).vi"("ISOBUS address"=w11, "error in"=w80, "Mercury Reference In"=w81) -> ("error out"=w78:errorcluster, "Unit"=→"Unit 6":T2, "Gear"=→"Gear":u32, "Mercury Reference Out"=w79:T26)  [unwired: 5 out]
  n47 = call-poly <instrlib>:"Configuration (Read).vi"("ISOBUS address"=w11, "error in"=w47, "Mercury Reference In"=w48) -> ("error out"=w181:errorcluster, "Serial Number"=→"Serial Number":string, "Mercury Reference Out"=w182:T26)  [unwired: 6 out]
  n48 = call-poly <instrlib>:"Signals (Read).vi"("ISOBUS address"=w11, "error in"=w150, "Mercury Reference In"=w151) -> ("error out"=w146:errorcluster, "Unit"=→"V Unit":T2, "Current"=→"Voltage":dbl, "Mercury Reference Out"=w147:T26)  [unwired: 5 out]
  n49 = call-poly <instrlib>:"Signals (Read).vi"("ISOBUS address"=w11, "error in"=w124, "Mercury Reference In"=w125) -> ("error out"=w122:errorcluster, "Unit"=→"Htr V Unit":T2, "Voltage"=→"Htr Voltage":dbl, "Mercury Reference Out"=w123:T26)  [unwired: 5 out]
  n50 = call-poly <instrlib>:"Configuration (Read).vi"("ISOBUS address"=w11, "error in"=w78, "Mercury Reference In"=w79) -> ("error out"=w64:errorcluster, "Unit"=→"Unit 7":T2, "Speed"=→"Speed":u32, "Mercury Reference Out"=w65:T26)  [unwired: 5 out]
  n51 = call-poly <instrlib>:"Signals (Read).vi"("ISOBUS address"=w11, "error in"=w146, "Mercury Reference In"=w147) -> ("error out"=w145:errorcluster, "Unit"=→"T Unit":T2, "Temperature"=→"Temperature":dbl, "Mercury Reference Out"=w141:T26)  [unwired: 5 out]
  n52 = call-poly <instrlib>:"Configuration (Read).vi"("ISOBUS address"=w11, "error in"=w181, "Mercury Reference In"=w182) -> ("error out"=w110:errorcluster, "Free Space"=→"Free Space":i32, "Mercury Reference Out"=w111:T26)  [unwired: 6 out]
  n53 = call-poly <instrlib>:"Signals (Read).vi"("ISOBUS address"=w11, "error in"=w122, "Mercury Reference In"=w123) -> ("error out"=w120:errorcluster, "Unit"=→"Htr P Unit":T2, "Power"=→"Htr Power":dbl, "Mercury Reference Out"=w121:T26)  [unwired: 5 out]
  n54 = call-poly <instrlib>:"Signals (Read).vi"("ISOBUS address"=w11, "error in"=w64, "Mercury Reference In"=w65) -> ("error out"=w62:errorcluster, "Unit"=→"Unit":T2, "Position"=→"Position":u32, "Mercury Reference Out"=w63:T26)  [unwired: 5 out]
  n55 = call-poly <instrlib>:"Configuration (Read).vi"("ISOBUS address"=w11, "error in"=w145, "Mercury Reference In"=w141) -> ("error out"=w97:errorcluster, "Device Details"=→"Temperature Device Settings":T3, "Mercury Reference Out"=w98:T26)  [unwired: 6 out]
  n56 = call-poly <instrlib>:"Configuration (Read).vi"("ISOBUS address"=w11, "error in"=w110, "Mercury Reference In"=w111) -> ("error out"=w176:errorcluster, "Mode"=→"String":T28, "Mercury Reference Out"=w175:T26)  [unwired: 6 out]
  n57 = call-poly <instrlib>:"Signals (Read).vi"("ISOBUS address"=w11, "error in"=w120, "Mercury Reference In"=w121) -> ("error out"=w16:errorcluster, "Unit"=→"Htr C Unit":T2, "Current"=→"Htr Current":dbl)  [unwired: 6 out]
  n58 = call-poly <instrlib>:"Signals (Read).vi"("ISOBUS address"=w11, "error in"=w62, "Mercury Reference In"=w63) -> ("error out"=w14:errorcluster, "Unit"=→"Unit":T2, "% Open"=→"% Open":dbl)  [unwired: 6 out]
  n59 = Get Date/Time In Seconds() -> (seconds since 1Jan1904=w49:timestamp)
  n60 = call-poly <instrlib>:"Configuration (Read).vi"("ISOBUS address"=w11, "error in"=w97, "Mercury Reference In"=w98) -> ("error out"=w17:errorcluster, "Loop Details"=→"T Loop Details":T10)  [unwired: 7 out]
  n61 = call-poly <instrlib>:"Configuration (Set).vi"("ISOBUS address"=w11, "error in"=w176, "time stamp"=w49, "Mercury Reference In"=w175) -> ("error out"=w18:errorcluster, "Response"=→"Set Date Response":T29, "Mercury Reference Out"=w42:T26)  [unwired: 5 out]
  n62 = Merge Errors(w18, w17, w16, w15, w14, w10) -> (w142:errorcluster)
  n63 = call <instrlib>:"Close.vi"("error in (no error)"=w142, "Mercury Reference"=w42) -> ("error out"=w52:errorcluster)  [unwired: 9 out]
  n64 = call <vilib>:"Simple Error Handler.vi"("error in (no error)"=w52) -> ()  [unwired: 1 in, 8 out]
